vi "JKI StateMachine 2024 ParseStatesAndLog.vi"   [LabVIEW 2020]
uses:
  <vilib>/MNProjects/Logging/Logging.lvlib
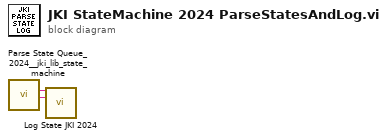
[diagram p0: block diagram]
diagram:
  n1 = call <vilib>:"Parse State Queue_2024__jki_lib_state_machine.vi"() -> ("Current State"=w2:string, "Arguments"=w1:string)  [unwired: 13 in, 1 out]
  n2 = call <vilib>:"Log State JKI 2024.vi"("Current State In"=w2, "Arguments In"=w1) -> ()  [unwired: 12 in, 2 out]
